vi "OSICS_Set_ESE.vi"(8 "error in (no error)":errorcluster, 11 "VISA resource name":refnum<visa-resource-name>) -> (0 "error out":errorcluster, 3 "VISA resource name out":refnum<visa-resource-name>)   [LabVIEW 2014, in "OSICS_LIB.lvlib"]
doc: "This Vi allows for the configuration settings of the Error Handling and Synchronisation registers of OSICS.\n\n Default value is SRE 56"
uses:
  OSICS_LIB.lvlib
panel:
  # "Basic function to configure the settings of the\nError handling registers of the OSICS"
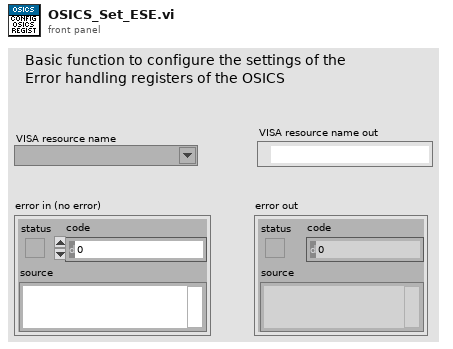
[diagram p1: front panel]
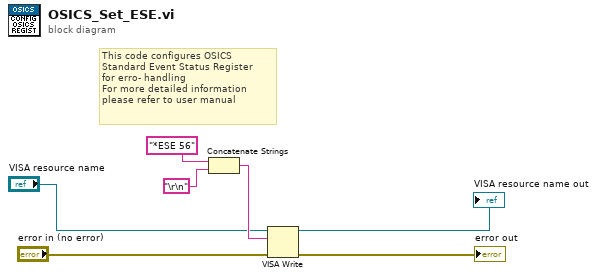
[diagram p0: block diagram]
diagram:
  # "This code configures OSICS\nStandard Event Status Register\nfor erro- handling \nFor more detailed information \nplease refer to user manual"
  n1 = Concatenate Strings("*ESE 56" ("string"), "\r\n") -> (w5:string)
  n2 = VISA Write(VISA resource name="VISA resource name", write buffer=w5, error in (no error)="error in (no error)") -> (VISA resource name out=→"VISA resource name out":refnum<visa-resource-name>, error out=→"error out":errorcluster)  [unwired: 1 out]
